vi "ArrayFunctions_CropArray(SGL).vi"(8 "length":i32, 11 "input array":sgl[](array[numeric])) -> (3 "output array":sgl[](array[numeric]))   [LabVIEW 2016]
doc: "Crops array to the last n elements, where n is the specified length.\n\nIf Array is shorter than specified length, does nothing.\n\nME 05 05 2015"
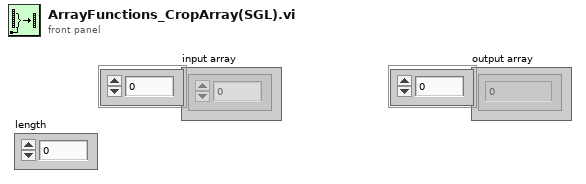
[diagram p1: front panel]
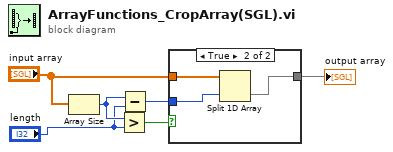
[diagram p0: block diagram]
diagram:
  n1 = Array Size(array="input array") -> (size(s)=w5:i32)
  n2 = Greater?(x=w5, y="length") -> (0:w6:bool)
  n3 = Subtract(x=w5, y="length") -> (x-y=w3:i32)
  n4 = case shown="True" w6 {
    tunnel: "input array" -> [w7 w10]
    tunnel: [w7 w9] -> w1
    tunnel: w3 -> [_ w8]
    frame False {
    }
    frame True {
      n5 = Split 1D Array(array=w10, index=w8) -> (second subarray=w9:sgl[])  [unwired: 1 out]
    }
  }
  "output array" <- w1
